vi "Extract Sentences.vi"(8 "error in (no error)":errorcluster, 9 "filter for sentence type":string, 10 "sensor data":string, 11 "previous partial sentence":string) -> (0 "error out":errorcluster, 2 "complete sentences":string[](array[string]), 3 "remaining partial sentence":string, 4 "invalid sentences":string[](array[string]), 5 "discarded data before first sentence":string)   [LabVIEW 2017, in "NMEA API.lvlib"]
doc: "Returns complete NMEA sentences contained in <B>sensor data</B>."
uses:
  <vilib>/robotics/Protocols/NMEA/NMEA API.lvlib
  <vilib>/regexp/Match Regular Expression.xnode
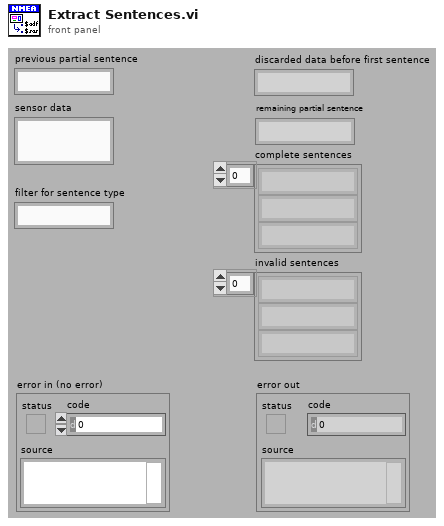
[diagram p1: front panel]
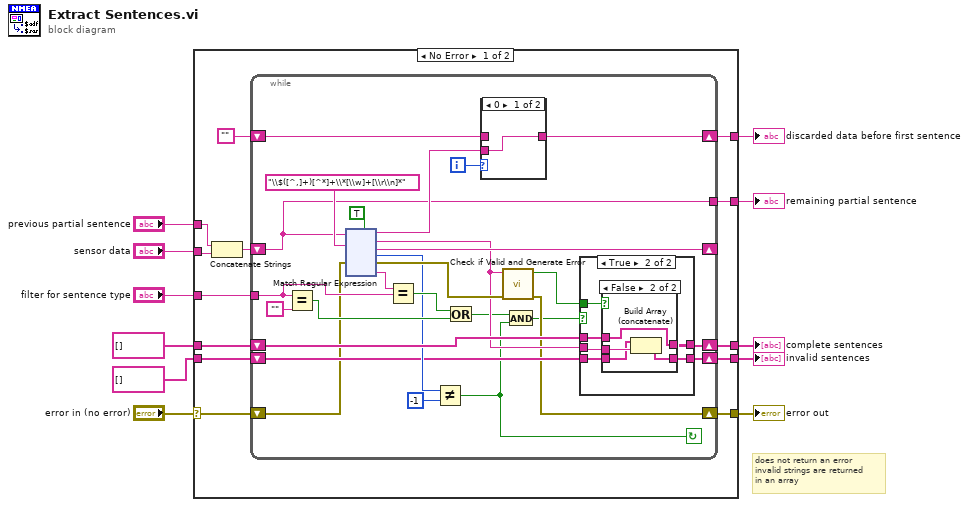
[diagram p0: block diagram]
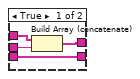
[diagram p3: hidden frame]
diagram:
  # "does not return an error\ninvalid strings are returned\nin an array"
  n1 = case shown="No Error" "error in (no error)" {
    selector: "error in (no error)" -> [w18 w185]
    tunnel: [w17 w185] -> w10
    tunnel: "previous partial sentence" -> [w14 _]
    tunnel: [w21 _] -> w8
    tunnel: "filter for sentence type" -> [w24 _]
    tunnel: "sensor data" -> [w15 _]
    tunnel: string[] [] -> [w23 w184]
    tunnel: [w22 w184] -> w4
    tunnel: string[] [] -> [w20 w183]
    tunnel: [w19 w183] -> w2
    tunnel: [w12 _] -> w1
    frame No Error {
      n2 = Concatenate Strings(w14, w15) -> (w16:string)
      n3 = while {
        tunnel: w24 -> [w44]
        shift-right: [w39] -> w22
        shift-left: w23 -> [w41]
        shift-right: [w48] -> _
        shift-left: w16 -> [w28]
        tunnel: [w28] -> w21
        shift-right: [w33] -> w19
        shift-left: w20 -> [w34]
        shift-right: [w31] -> w17
        shift-left: w18 -> [w32]
        shift-right: [w25] -> w12
        shift-left: "" -> [w26]
        i -> [w51]
        stop <- w29 continue-if-true
        n4 = Equal?(x=w44, y="") -> (x = y?=w42:bool)
        n5 = xnode "Match Regular Expression"("input string"=w28, "regular expression"="\\$([^,]+)[^*]+\\*[\\w]+[\\r\\n]*", "error in"=w32, "multiline? (F)"=TRUE) -> ("before match"=w49:string, "whole match"=w40:string, "after match"=w48:string, "offset past match"=w38:i32, "error out"=w47:errorcluster, "submatch 1"=w45:string)  [unwired: 1 in, 1 out]
        n6 = Equal?(x=w45, y=w44) -> (x = y?=w43:bool)
        n7 = Not Equal?(x=w38, y=-1) -> (x != y?=w29:bool)
        n8 = Or(x=w43, y=w42) -> (x .or. y?=w36:bool)
        n9 = case shown="0" w51 {
          tunnel: w49 -> [w68 _]
          tunnel: w26 -> [_ w69]
          tunnel: [w68 w69] -> w25
          frame 0 {
          }
          frame 1, Default {
          }
        }
        n10 = call <vilib>:"Check if Valid and Generate Error.vi"("error in (no error)"=w47, "sentence"=w40) -> ("error out"=w31:errorcluster, "valid sentence"=w35:bool)  [unwired: 8 in]
        n11 = And(x=w36, y=w29) -> (x .and. y?=w30:bool)
        n12 = case shown="True" w30 {
          tunnel: w41 -> [w53 w59]
          tunnel: w40 -> [_ w58]
          tunnel: [w53 w57] -> w39
          tunnel: w35 -> [_ w56]
          tunnel: w34 -> [w52 w55]
          tunnel: [w52 w54] -> w33
          frame False {
          }
          frame True {
            n13 = case shown="False" w56 {
              tunnel: w59 -> [w63 w64]
              tunnel: w58 -> [w62 w67]
              tunnel: [w61 w64] -> w57
              tunnel: w55 -> [w60 w66]
              tunnel: [w60 w65] -> w54
              frame True {
                n14 = Build Array (concatenate)(w63, w62) -> (w61:string[])
              }
              frame False {
                n15 = Build Array (concatenate)(w66, w67) -> (w65:string[])
              }
            }
          }
        }
      }
    }
    frame Error {
    }
  }
  "complete sentences" <- w4
  "remaining partial sentence" <- w8
  "error out" <- w10
  "invalid sentences" <- w2
  "discarded data before first sentence" <- w1
